vi "Get or Add TableParts.vi"(7 "Sheet Name":string, 8 "error in":errorcluster, 11 "SpreadsheetDoc in":refnum<k24>) -> (0 "error out":errorcluster, 2 "TableParts":refnum<k24>, 3 "SpreadsheetDoc out":refnum<k24>, 5 "Sheet Name":string)   [LabVIEW 2019, in "Open Xml.lvlib"]
uses:
  Open Xml.lvlib
  D:/git/Open-Xml-LabVIEW/Source/DocumentFormat.OpenXml.dll
  DocumentFormat.OpenXml.dll
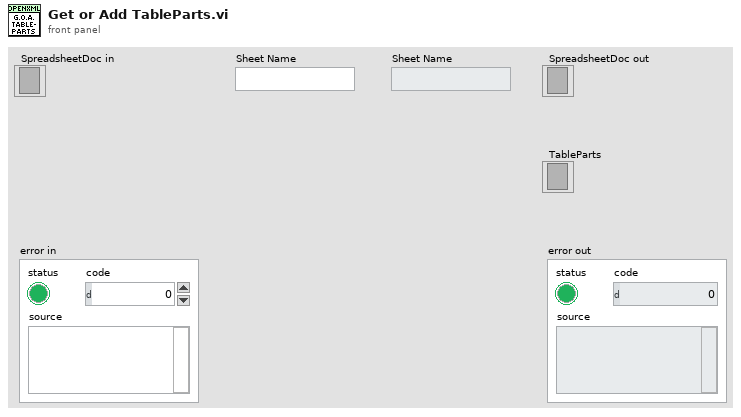
[diagram p1: front panel]
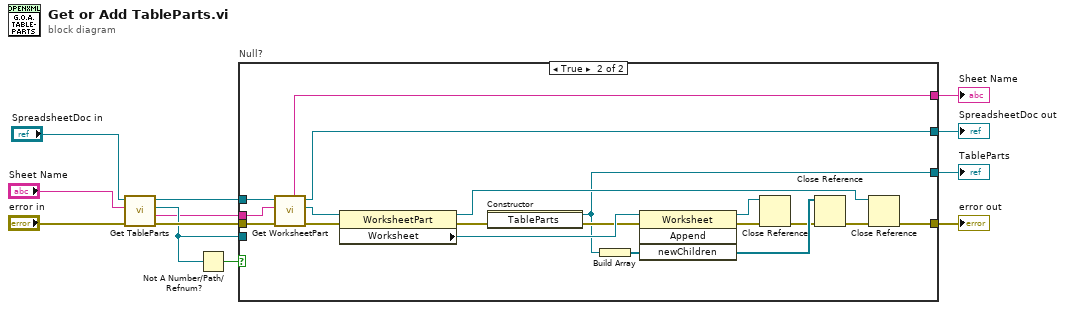
[diagram p0: block diagram]
diagram:
  n1 = call "Get TableParts.vi"("error in"="error in", "Sheet Name"="Sheet Name", "SpreadsheetDoc in"="SpreadsheetDoc in") -> ("error out"=w6:errorcluster, "SheetName"=w3:string, "TableParts"=w5:refnum<k24>, "SpreadsheetDoc out"=w4:refnum<k24>)  [unwired: 5 in]
  n2 = Not A Number/Path/Refnum?(number/path/refnum=w5) -> (NaN/Path/Refnum?=w9:bool)
  n3 = case "Null?" shown="True" w9 {
    tunnel: w5 -> [w16 _]
    tunnel: w6 -> [w15 w35]
    tunnel: [w15 w21] -> w7
    tunnel: [w16 w17] -> w8
    tunnel: w4 -> [w14 w33]
    tunnel: w3 -> [w13 w34]
    tunnel: [w13 w32] -> w2
    tunnel: [w14 w19] -> w1
    frame False {
    }
    frame True {
      n4 = call "Get WorksheetPart.vi"("error in"=w35, "Sheet Name"=w34, "SpreadsheetDoc in"=w33) -> ("error out"=w31:errorcluster, "WorksheetPart"=w30:refnum<k24>, "SpreadsheetDoc out"=w19:refnum<k24>, "SheetName"=w32:string)  [unwired: 5 in]
      n5 = property class="WorksheetPart"(reference=w30, error in=w31) -> (reference out=w20:refnum<k24>, error out=w28:errorcluster, "Worksheet"=w29:refnum<k24>)
      n6 = constructor class="TableParts"(error in=w28) -> (reference out=w17:refnum<k24>, error out=w27:errorcluster)  [unwired: 2 in, 1 out]
      n7 = Build Array(w17) -> (w22:refnum<k24>[])
      n8 = invoke class="Worksheet" method="Append"(reference=w29, error in=w27, "newChildren"=w22) -> (reference out=w23:refnum<k24>, error out=w26:errorcluster, "newChildren"=w25:refnum<k24>[])  [unwired: 1 in, 1 out]
      n9 = Close Reference(reference=w23, error in (no error)=w26) -> (error out=w24:errorcluster)
      n10 = Close Reference(reference=w25, error in (no error)=w24) -> (error out=w18:errorcluster)
      n11 = Close Reference(reference=w20, error in (no error)=w18) -> (error out=w21:errorcluster)
    }
  }
  "error out" <- w7
  "SpreadsheetDoc out" <- w1
  "TableParts" <- w8
  "Sheet Name" <- w2
